vi "MeasurementGFV.vi"(8 "error in (no error)":errorcluster, 10 "MeasuremetnGFVEnum":T1=enum."Insert Single Measurement", 11 "Variant in":variant) -> (0 "error out":errorcluster, 3 "Variant Out":variant)   [LabVIEW 2013]
doc: "Use this template to build a VI to use as a subVI."
uses:
  Measurement Typedefs/MeasurementGFV.ctl
  General TypeDefs/MeasurementType.ctl
  General TypeDefs/ConfigurationDataTypeDef.ctl
  General TypeDefs/MeasurementDataType.ctl
  <vilib>/Utility/file.llb/Write To Spreadsheet File (string).vi
  Measurement Typedefs/KineticNotifierDatatype.ctl
panel:
  out "size(s)":i32
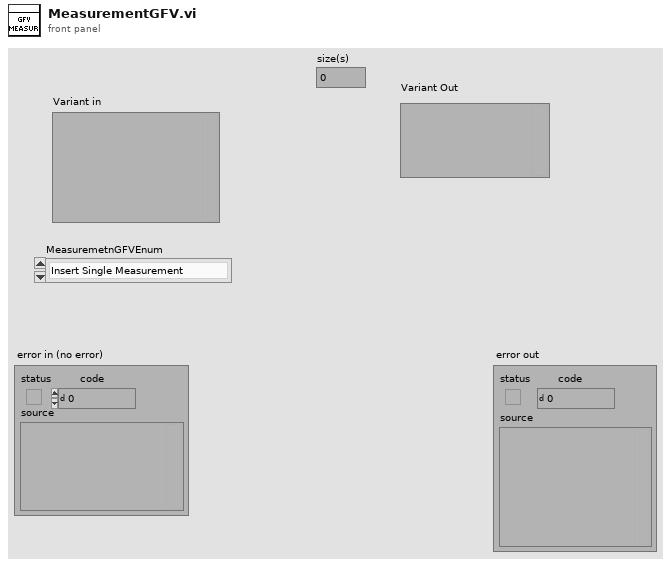
[diagram p1: front panel]
types:
  T1 = typedef "MeasurementGFV.ctl" = enum16{"Write 2 Excel", "Open Excel", "Close Excel", "Export To Excel", "GetExperimentGoalRemarks", "Load Single DB", "Save Single 2 DB", "Load Kinetic DB", "Save Kinetic 2 DB", "Get List of Wavelength", "Remove Wavelength", "Add Wavelength", "Get Sample Names", "Insert Sample Name", "Update Kinetic Display", "Update Single Display", "Init", "Insert General", "Init Single Measurement", "Insert Single Measurement", "Insert Kinetic Measurement", "Init Kinetic Measurment", "Init General"}
  T2 = typedef "MeasurementType.ctl" = enum16{"Single Meas", "Kinetic"}
  T3 = enum16{"open", "replace", "create", "open or create", "replace or create", "replace or create with confirmation"}
  T4 = typedef "ConfigurationDataTypeDef.ctl" = cluster{"Experiment Name":string, "File Path":path, "Goal":string, "Remarks":string, "Time Between Consecutive Frames (sec)":dbl, "Rq. No. of saves":i32, "Enable\nAutomatic\nStop":bool, "Measurement Type":T2, "File Name":string, "Choose Spectrometer":refnum<visa-resource-name>, "Integration time (ms)":i32, "Delay between measurements (ms) ":i32, "Offset in Wavlength (nm)":dbl}
  T5 = typedef "MeasurementDataType.ctl" = cluster{"Wavelength (nm)":dbl[], "Absorption":dbl[][], "Time":timestamp[], "Ref Spectrum":dbl[], "Dark Spectrum":dbl[], "Number of\nsamples to average":i32, "Measured Spectrum":dbl[][], "Sample Name":string[], "Selected Wavelengths":dbl[]}
  T6 = cluster{"General Data and Instrument Configuration":T4, "Kinetic Measurement":T5}
  T7 = cluster{"Absorption Saved Results":refnum<vi>, "Absorption @ wavelengths vs Time":refnum<vi>, "Selected Wavelengths":refnum<vi>}
  T8 = typedef "NI_Matrix.lvlib/RealMatrix.ctl" = dbl[][]
  T9 = cluster{"Experiment Name":string, "Goal":string, "Remarks":string, "File Path":path}
  T10 = cluster{"Wavelength (nm)":dbl[], "Absorption":dbl[]}
  T11 = cluster{"Wavelength (nm)":dbl[], "Absorption":dbl[]}[]
  T12 = typedef "KineticNotifierDatatype.ctl" = cluster{"Wavelength (nm)":dbl[], "Dark_spectrum":dbl[], "Meas_spectrum":dbl[], "Ref_spectrum":dbl[], "Absorption_spectrum":dbl[]}
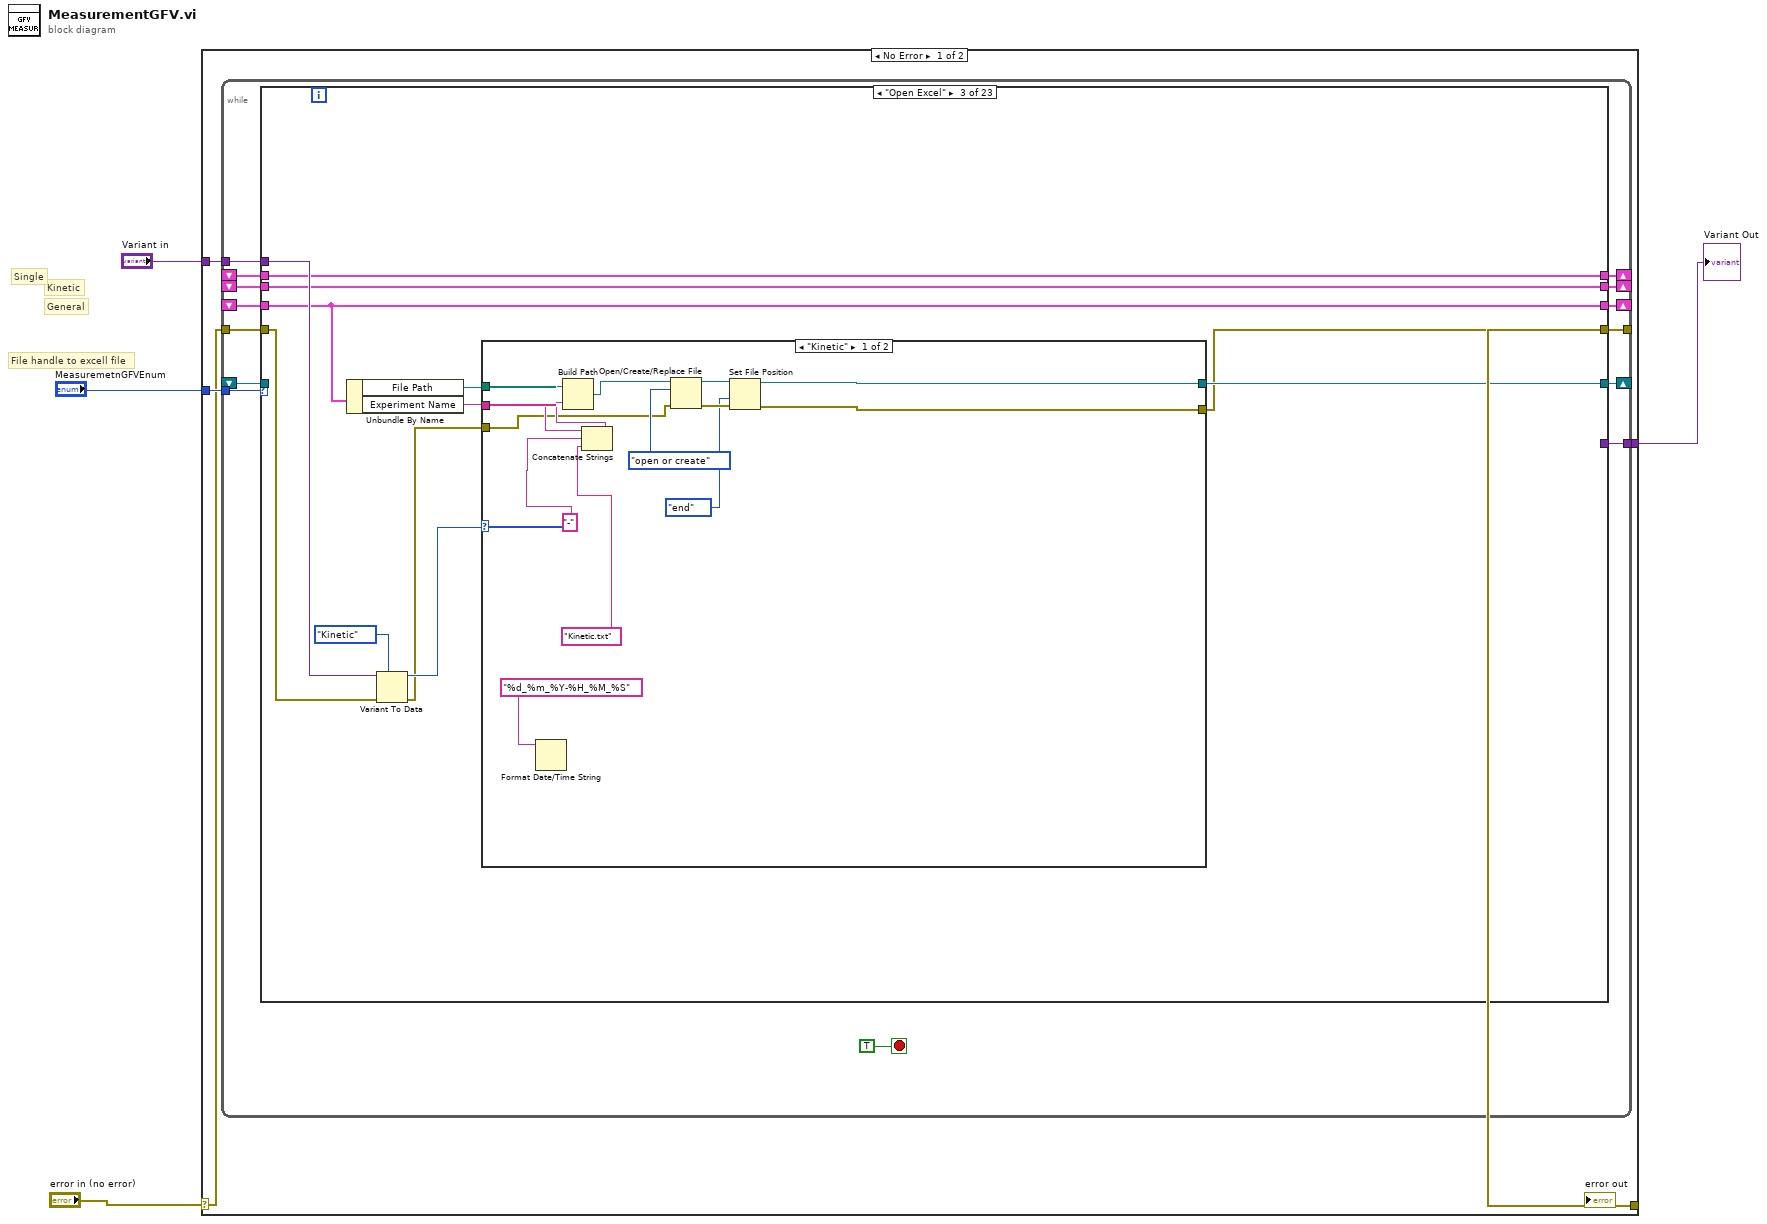
[diagram p0: block diagram]
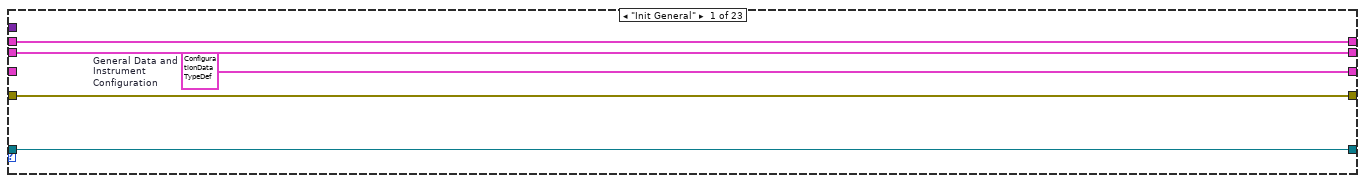
[diagram p2: hidden frame]
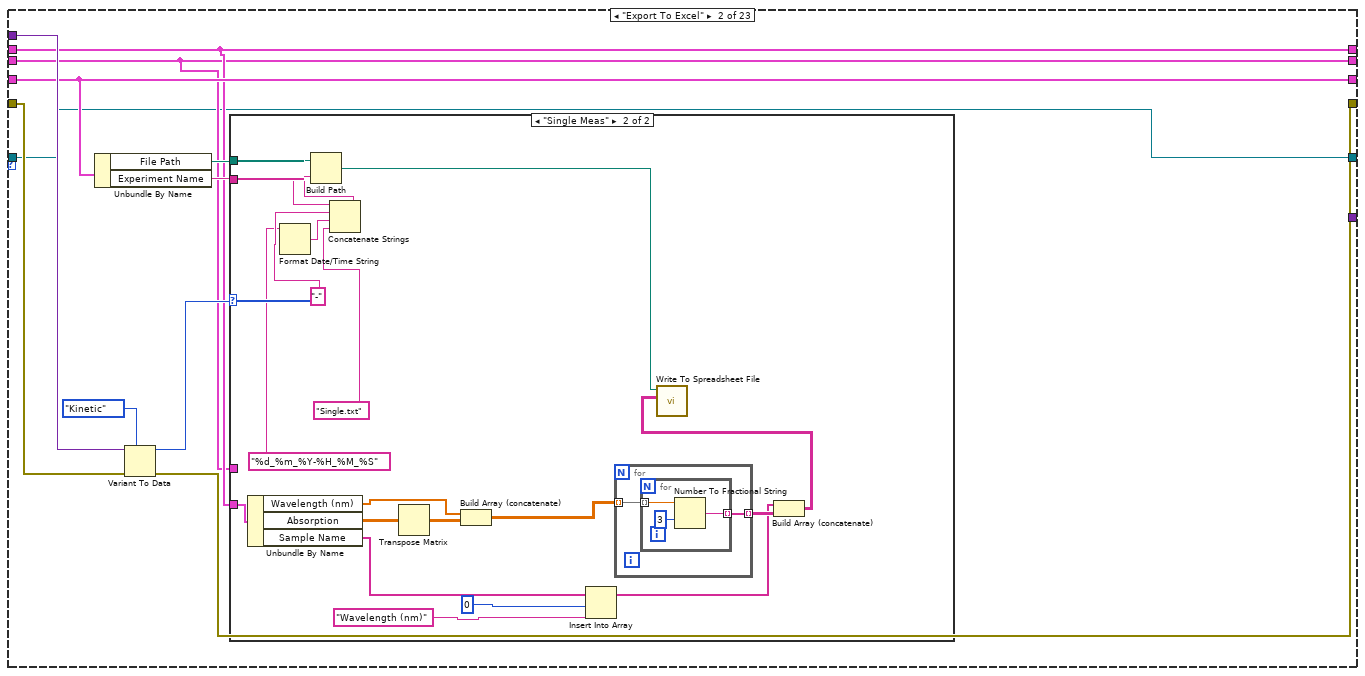
[diagram p3: hidden frame]
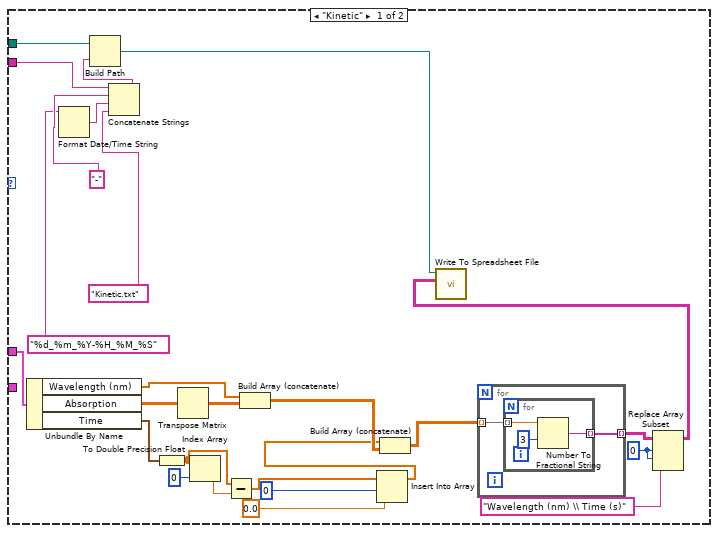
[diagram p4: hidden frame]
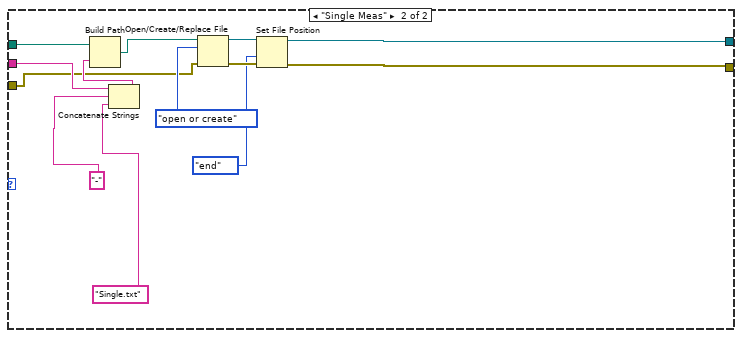
[diagram p5: hidden frame]
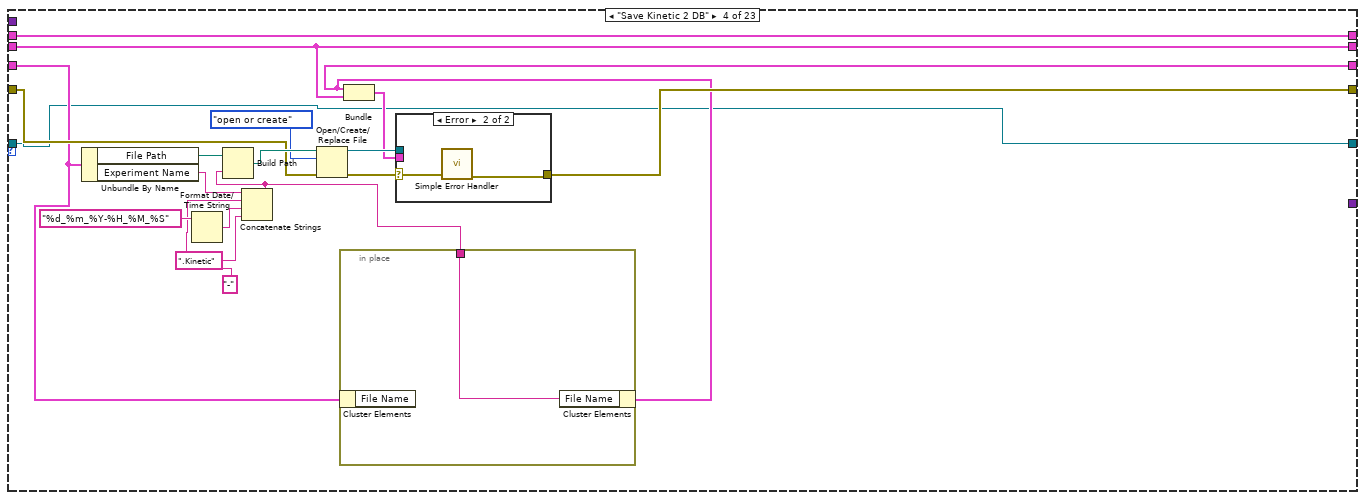
[diagram p6: hidden frame]
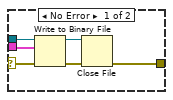
[diagram p7: hidden frame]
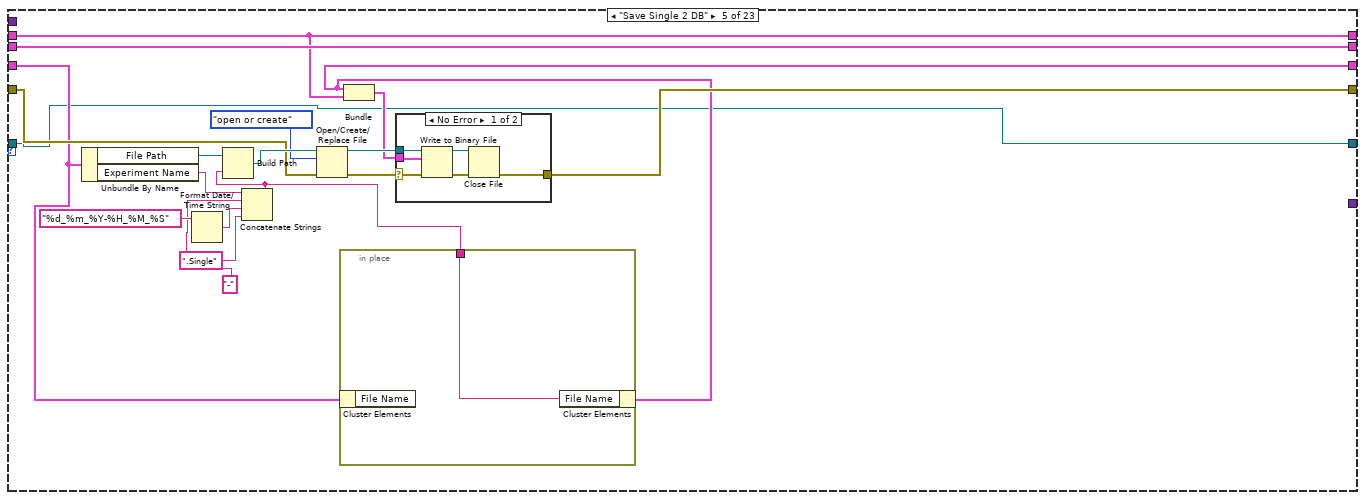
[diagram p8: hidden frame]
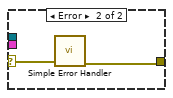
[diagram p9: hidden frame]
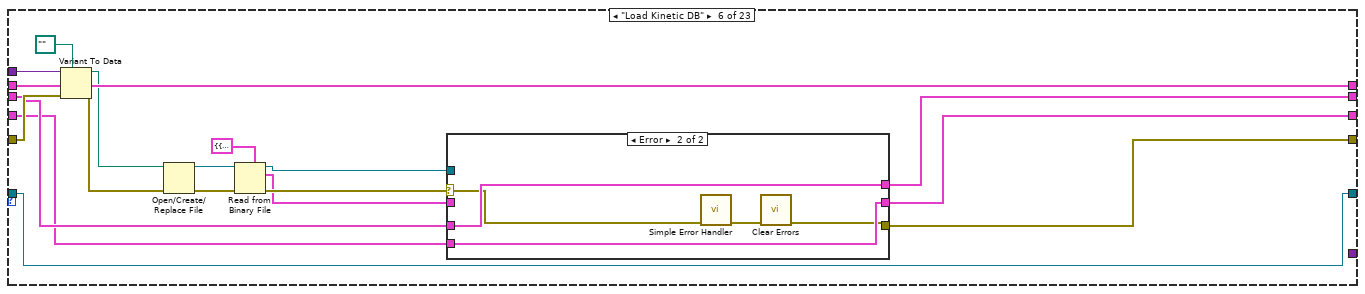
[diagram p10: hidden frame]
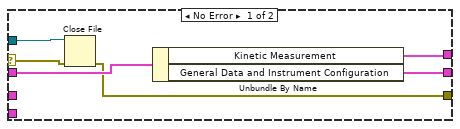
[diagram p11: hidden frame]
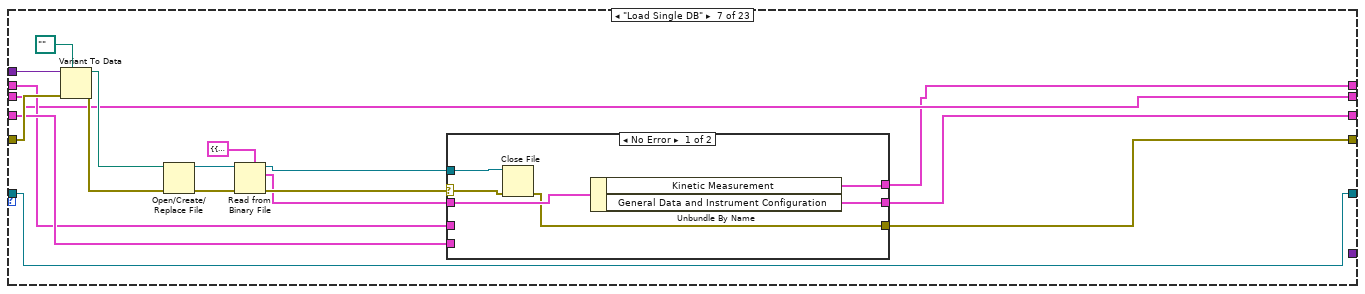
[diagram p12: hidden frame]
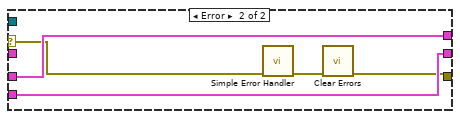
[diagram p13: hidden frame]
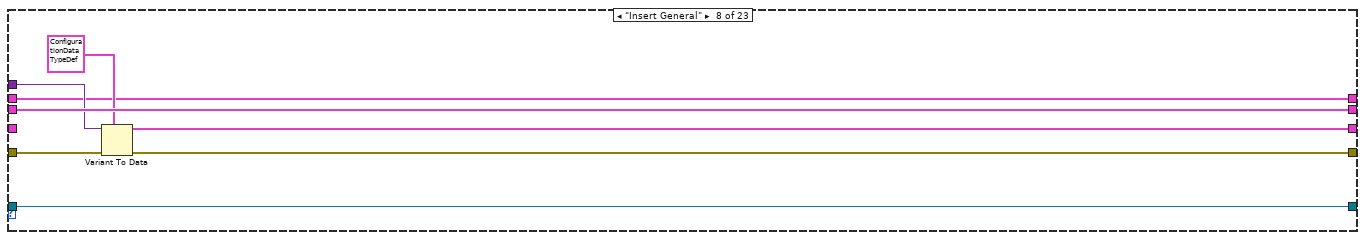
[diagram p14: hidden frame]
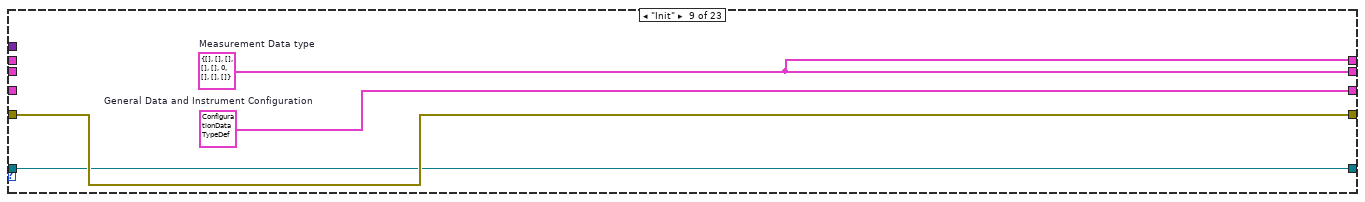
[diagram p15: hidden frame]
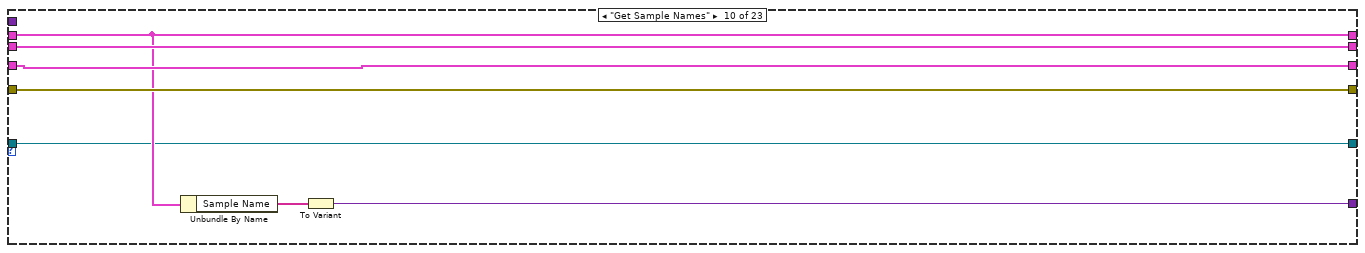
[diagram p16: hidden frame]
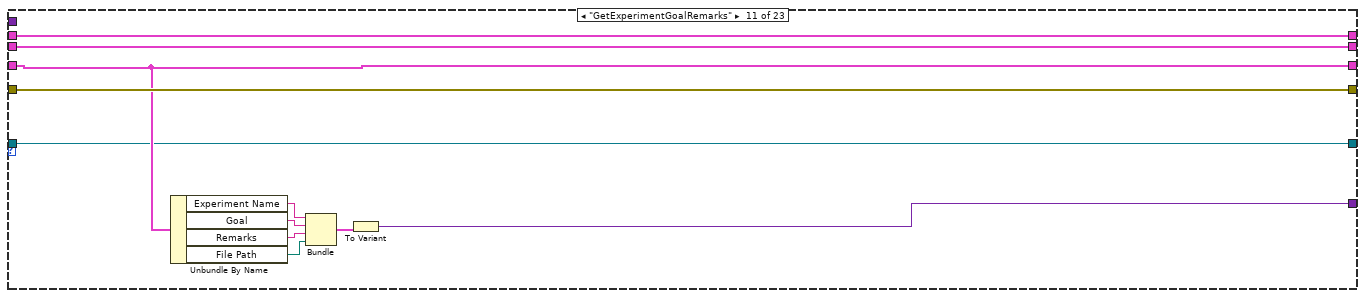
[diagram p17: hidden frame]
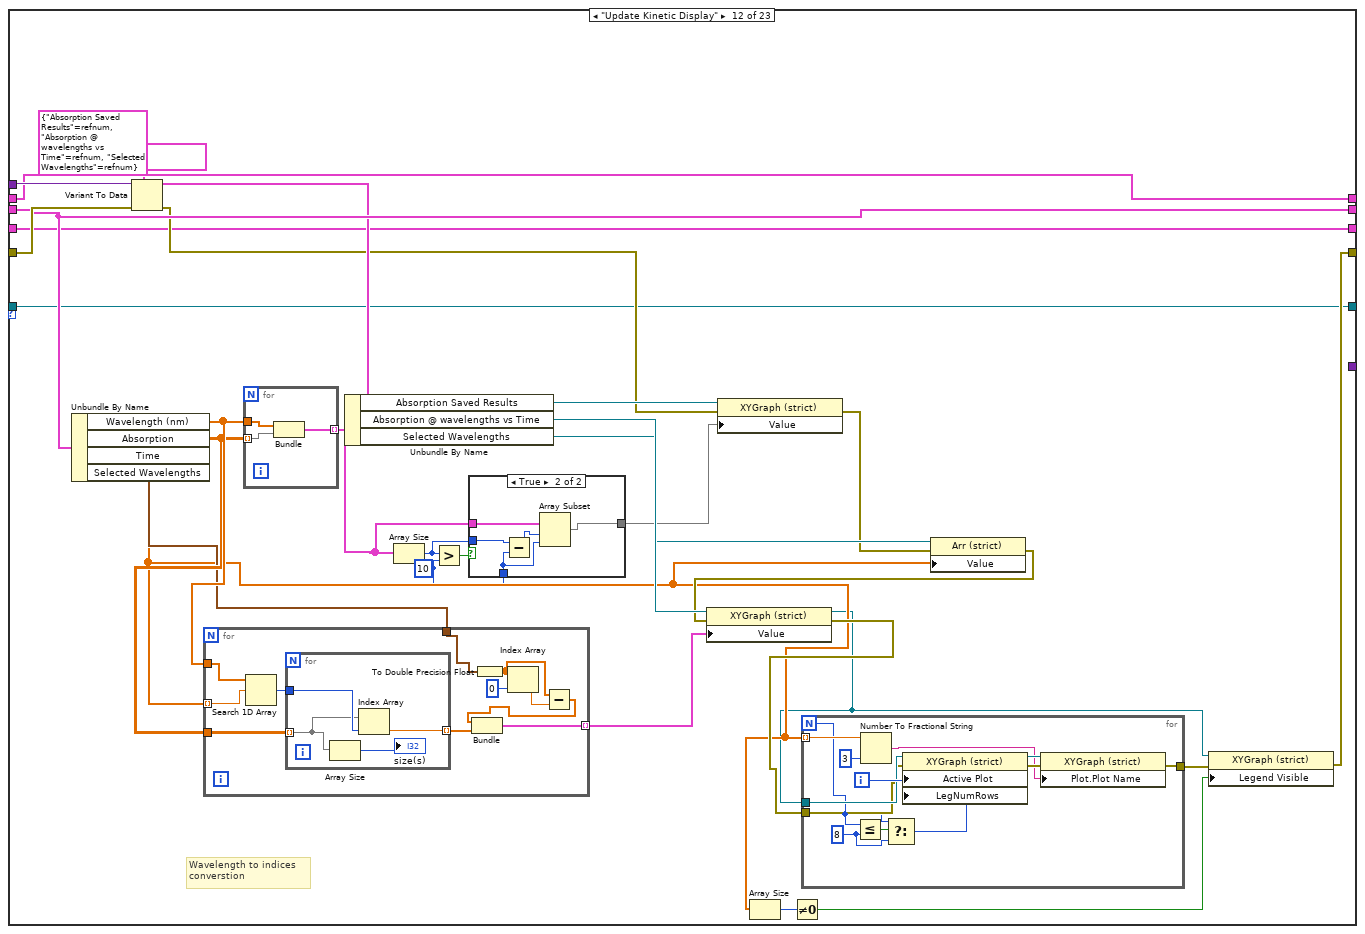
[diagram p18: hidden frame]
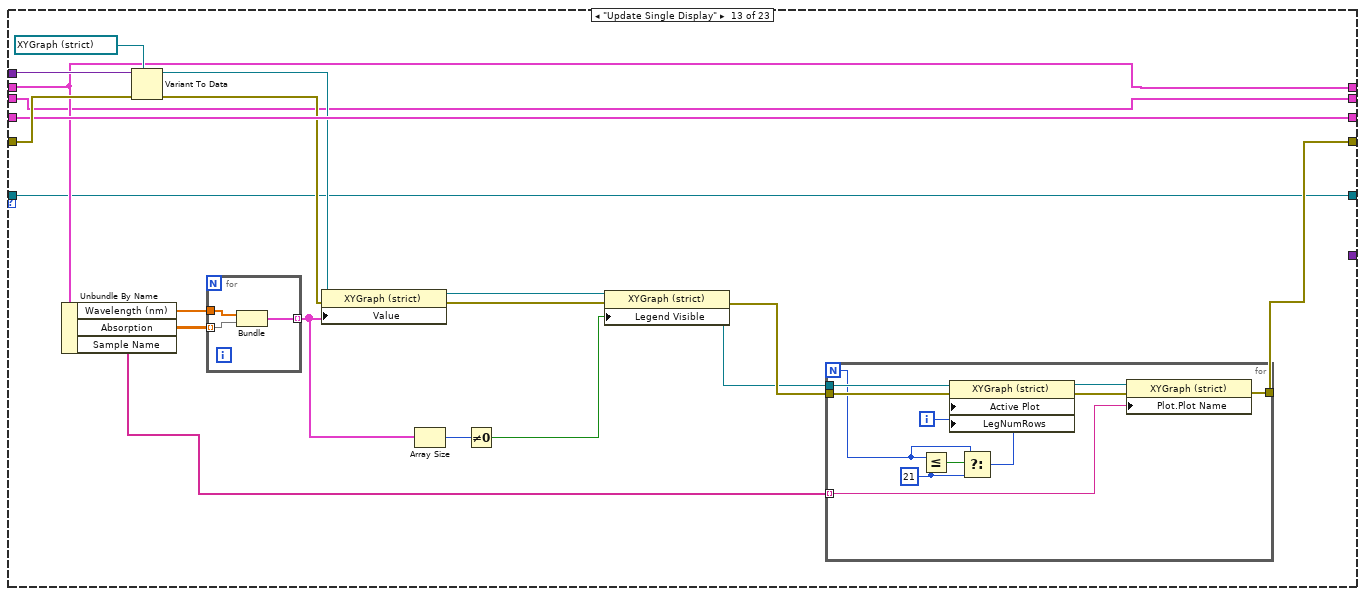
[diagram p20: hidden frame]
diagram:
  # "File handle to excell file"
  # "Single"
  # "General"
  # "Kinetic"
  n1 = case shown="No Error" "error in (no error)" {
    selector: "error in (no error)" -> [w8 w590]
    tunnel: [w7 w590] -> w4
    tunnel: "Variant in" -> [w10 _]
    tunnel: "MeasuremetnGFVEnum" -> [w9 _]
    tunnel: [w6 _] -> w1
    frame No Error {
      n2 = while {
        tunnel: w10 -> [w18]
        tunnel: w9 -> [w23]
        shift-right: [w22] -> _
        shift-left: _ -> [w20]
        shift-right: [w21] -> _
        shift-left: _ -> [w19]
        tunnel: w8 -> [w17]
        tunnel: [w16] -> w7
        shift-right: [w15] -> _
        shift-left: _ -> [w14]
        tunnel: [w13] -> w6
        shift-right: [w12] -> _
        shift-left: _ -> [w11]
        stop <- TRUE stop-if-true
        n3 = case shown="\"Open Excel\"" w23 {
          tunnel: [w28 w31 w99 w141 w170 w196 w222 w256 w258 w265 w277 w306 w355 w381 w396 w402 w415 w426 w447 w469 w478 w488 w490] -> w22
          tunnel: [w29 w37 w104 w136 w165 w195 w227 w253 w260 w266 w274 w296 w363 w389 w399 w401 w416 w432 w454 w474 w481 w487 w500] -> w21
          tunnel: w20 -> [w28 w31 w99 w141 w170 w193 w222 w256 _ w265 w277 w306 w355 w381 w396 w403 w414 w428 w447 w470 w478 w488 w490]
          tunnel: w19 -> [_ w37 w104 w138 w167 w192 w225 _ _ w266 w274 w296 w363 w389 w399 w401 w416 w432 w454 w474 w481 w487 w500]
          tunnel: w18 -> [_ w40 w107 _ _ w207 w237 w255 _ _ _ w308 w365 w388 _ w409 _ w429 w451 _ _ _ w498]
          tunnel: w17 -> [w27 w39 w106 w144 w173 w206 w236 w252 w259 w267 w278 w307 w364 w387 w397 w408 w417 w431 w453 w473 w480 w485 w497]
          tunnel: [w27 w33 w96 w142 w171 w194 w226 w251 w259 w267 w278 w285 w354 w386 w397 w407 w417 w431 w453 w473 w480 w482 w492] -> w16
          tunnel: [w26 w32 w100 w153 w164 w208 w221 w250 w258 w264 w276 w302 w356 w382 w398 w405 w418 w425 w448 w472 w479 w489 w491] -> w15
          tunnel: w14 -> [w26 w32 w100 w153 w164 w208 w223 w250 _ w264 w276 w302 w356 w383 w398 w405 w418 w425 w449 w472 _ w489 w491]
          tunnel: [_ _ _ _ _ _ _ _ _ w262 w275 _ _ _ w394 _ _ _ _ _ _ _ _] -> w13
          tunnel: [w25 w30 w98 w135 w163 w191 w220 w249 w257 w261 w269 w284 w346 w380 w393 w400 w413 w424 w446 w468 w477 refnum<file> refnum ("refnum out") w494] -> w12
          tunnel: w11 -> [w25 w30 _ w135 w163 w191 w220 w249 w257 w261 w269 w284 w346 w380 w393 w400 w413 w424 w446 w468 w477 w486 w495]
          frame "Init General" {
            w29 = T4 {"Experiment Name"="", "File Path"=path "E:/LINKAM Measurements_Naama", "Goal"="", "Remarks"="", "Time Between Consecutive Frames (sec)"=1.0, "Rq. No. of saves"=1, "Enable\nAutomatic\nStop"=TRUE, "Measurement Type"=enum."Single Meas", "File Name"="", "Choose Spectrometer"="USB650", "Integration time (ms)"=49, "Delay between measurements (ms) "=10, "Offset in Wavlength (nm)"=10.0}  # General Data and Instrument Configuration
          }
          frame "Export To Excel" {
            n4 = Unbundle By Name(w37) -> ("File Path"=w36:path, "Experiment Name"=w35:string)
            n5 = Variant To Data(error in=w39, type=MeasurementType."Kinetic" ("Measurement Type"), Variant=w40) -> (data=w34:T2, error out=w33:errorcluster)
            n6 = case shown="\"Single Meas\"" w34 {
              tunnel: w36 -> [w61 w85]
              tunnel: w35 -> [w60 w84]
              tunnel: w32 -> [_ w83]
              tunnel: w31 -> [w41 _]
              frame "Kinetic" {
                w44 = 0 ("index (row)")
                n7 = Unbundle By Name(w41) -> ("Wavelength (nm)"=w58:dbl[], "Absorption"=w59:dbl[][], "Time"=w52:timestamp[])
                n8 = Format Date/Time String(time format string (%c)="%d_%m_%Y-%H_%M_%S") -> (date/time string=w65:string)  [unwired: 2 in]
                n9 = Concatenate Strings(w60, "-" ("string"), w65, "Kinetic.txt" ("string")) -> (w66:string)
                n10 = Build Path(base path=w61, name or relative path=w66) -> (appended path=w56:path)
                n11 = To Double Precision Float(number=w52) -> (double precision float=w54:dbl[])
                n12 = Transpose Matrix(1:w59) -> (0:w57:dbl[][])
                n13 = Index Array(array=w54, index=0) -> (element=w53:dbl)
                n14 = Subtract(x=w54, y=w53) -> (x-y=w50:dbl[])
                n15 = Build Array (concatenate)(w58, w57) -> (w51:T8)
                n16 = Insert Into Array(array=w50, index=0, new element=0.0 ("new element/subarray")) -> (w47:dbl[])
                n17 = Build Array (concatenate)(w47, w51) -> (w46:T8)
                n18 = for {
                  tunnel: w46 -> [w68] mode=indexing
                  tunnel: [w67] -> w45 mode=indexing
                  n19 = for {
                    tunnel: w68 -> [w70] mode=indexing
                    tunnel: [w69] -> w67 mode=indexing
                    n20 = Number To Fractional String(number=w70, precision (6)=i16 3) -> (F-format string=w69:string)  [unwired: 2 in]
                  }
                }
                n21 = Replace Array Subset(array=w45, new element="Wavelength (nm) \\ Time (s)" ("new element/subarray"), index (row)=w44, index (col)=w44) -> (w42:string[][])
                n22 = call-poly <vilib>:"Write To Spreadsheet File.vi"("2D data"=w42, "file path (dialog if empty)"=w56) -> ()  [unwired: 6 in, 1 out]
              }
              frame "Single Meas" {
                n23 = Unbundle By Name(w83) -> ("Wavelength (nm)"=w81:dbl[], "Absorption"=w82:dbl[][], "Sample Name"=w77:string[])
                n24 = Format Date/Time String(time format string (%c)="%d_%m_%Y-%H_%M_%S") -> (date/time string=w89:string)  [unwired: 2 in]
                n25 = Concatenate Strings(w84, "-" ("string"), w89, "Single.txt" ("string")) -> (w90:string)
                n26 = Build Path(base path=w85, name or relative path=w90) -> (appended path=w79:path)
                n27 = Transpose Matrix(1:w82) -> (0:w80:dbl[][])
                n28 = Build Array (concatenate)(w81, w80) -> (w75:T8)
                n29 = Insert Into Array(array=w77, index=0, new element="Wavelength (nm)" ("new element/subarray")) -> (w73:string[])
                n30 = for {
                  tunnel: w75 -> [w92] mode=indexing
                  tunnel: [w91] -> w74 mode=indexing
                  n31 = for {
                    tunnel: w92 -> [w94] mode=indexing
                    tunnel: [w93] -> w91 mode=indexing
                    n32 = Number To Fractional String(number=w94, precision (6)=i16 3) -> (F-format string=w93:string)  [unwired: 2 in]
                  }
                }
                n33 = Build Array (concatenate)(w73, w74) -> (w72:string[][])
                n34 = call-poly <vilib>:"Write To Spreadsheet File.vi"("2D data"=w72, "file path (dialog if empty)"=w79) -> ()  [unwired: 6 in, 1 out]
              }
            }
          }
          frame "Open Excel" {
            n35 = Unbundle By Name(w104) -> ("File Path"=w103:path, "Experiment Name"=w102:string)
            n36 = Variant To Data(error in=w106, type=MeasurementType."Kinetic" ("Measurement Type"), Variant=w107) -> (data=w101:T2, error out=w97:errorcluster)
            n37 = case shown="\"Kinetic\"" w101 {
              tunnel: w103 -> [w118 w132]
              tunnel: w102 -> [w117 w131]
              tunnel: [w110 w124] -> w98
              tunnel: w97 -> [w111 w125]
              tunnel: [w109 w123] -> w96
              frame "Kinetic" {
                n38 = Format Date/Time String(time format string (%c)="%d_%m_%Y-%H_%M_%S") -> ()  [unwired: 2 in, 1 out]
                n39 = Concatenate Strings(w117, "-" ("string"), "Kinetic.txt" ("string")) -> (w121:string)
                n40 = Build Path(base path=w118, name or relative path=w121) -> (appended path=w116:path)
                n41 = Open/Create/Replace File(file path (use dialog)=w116, error in=w111, operation (0:open)=T3."open or create") -> (refnum out=w113:refnum<file>, error out=w114:errorcluster)  [unwired: 3 in, 1 out]
                n42 = Set File Position(refnum=w113, from (0:start)=enum16{"start", "end", "current"}."end", error in=w114) -> (refnum out=w110:refnum<file>, error out=w109:errorcluster)  [unwired: 1 in]
              }
              frame "Single Meas" {
                n43 = Concatenate Strings(w131, "-" ("string"), "Single.txt" ("string")) -> (w134:string)
                n44 = Build Path(base path=w132, name or relative path=w134) -> (appended path=w130:path)
                n45 = Open/Create/Replace File(file path (use dialog)=w130, error in=w125, operation (0:open)=T3."open or create") -> (refnum out=w127:refnum<file>, error out=w128:errorcluster)  [unwired: 3 in, 1 out]
                n46 = Set File Position(refnum=w127, from (0:start)=enum16{"start", "end", "current"}."end", error in=w128) -> (refnum out=w124:refnum<file>, error out=w123:errorcluster)  [unwired: 1 in]
              }
            }
          }
          frame "Save Kinetic 2 DB" {
            n47 = Unbundle By Name(w138) -> ("File Path"=w148:path, "Experiment Name"=w147:string)
            n48 = Format Date/Time String(time format string (%c)="%d_%m_%Y-%H_%M_%S") -> (date/time string=w150:string)  [unwired: 2 in]
            n49 = Concatenate Strings(w147, "-" ("string"), w150, ".Kinetic" ("string")) -> (w137:string)
            n50 = Build Path(base path=w148, name or relative path=w137) -> (appended path=w146:path)
            n51 = Open/Create/Replace File(file path (use dialog)=w146, error in=w144, operation (0:open)=T3."open or create") -> (refnum out=w143:refnum<file>, error out=w139:errorcluster)  [unwired: 3 in, 1 out]
            n52 = in-place {
              in-place-border: w137 -> [w154]
              n53 = in-place-cluster #1(w138) -> ()  [unwired: 1 out]
              n54 = in-place-cluster #1("File Name"=w154) -> (w136:T4)
            }
            n55 = Bundle("General Data and Instrument Configuration"=w136, "Kinetic Measurement"=w141) -> (w140:T6)  [unwired: 1 in]
            n56 = case shown="Error" w139 {
              selector: w139 -> [w155 w162]
              tunnel: w143 -> [w160 _]
              tunnel: [w157 w161] -> w142
              tunnel: w140 -> [w156 _]
              frame No Error {
                n57 = Write to Binary File(file (use dialog)=w160, data=w156, error in=w155) -> (refnum out=w158:refnum<file>, error out=w159:errorcluster)  [unwired: 3 in, 1 out]
                n58 = Close File(refnum=w158, error in=w159) -> (error out=w157:errorcluster)  [unwired: 1 out]
              }
              frame Error {
                n59 = call <vilib>:"Simple Error Handler.vi"("error in (no error)"=w162) -> ("error out"=w161:errorcluster)  [unwired: 4 in, 4 out]
              }
            }
          }
          frame "Save Single 2 DB" {
            n60 = Unbundle By Name(w167) -> ("File Path"=w177:path, "Experiment Name"=w176:string)
            n61 = Format Date/Time String(time format string (%c)="%d_%m_%Y-%H_%M_%S") -> (date/time string=w179:string)  [unwired: 2 in]
            n62 = Concatenate Strings(w176, "-" ("string"), w179, ".Single" ("string")) -> (w166:string)
            n63 = Build Path(base path=w177, name or relative path=w166) -> (appended path=w175:path)
            n64 = Open/Create/Replace File(file path (use dialog)=w175, error in=w173, operation (0:open)=T3."open or create") -> (refnum out=w172:refnum<file>, error out=w168:errorcluster)  [unwired: 3 in, 1 out]
            n65 = in-place {
              in-place-border: w166 -> [w182]
              n66 = in-place-cluster #2(w167) -> ()  [unwired: 1 out]
              n67 = in-place-cluster #2("File Name"=w182) -> (w165:T4)
            }
            n68 = Bundle("General Data and Instrument Configuration"=w165, "Kinetic Measurement"=w164) -> (w169:T6)  [unwired: 1 in]
            n69 = case shown="No Error" w168 {
              selector: w168 -> [w183 w190]
              tunnel: w172 -> [w188 _]
              tunnel: [w185 w189] -> w171
              tunnel: w169 -> [w184 _]
              frame No Error {
                n70 = Write to Binary File(file (use dialog)=w188, data=w184, error in=w183) -> (refnum out=w186:refnum<file>, error out=w187:errorcluster)  [unwired: 3 in, 1 out]
                n71 = Close File(refnum=w186, error in=w187) -> (error out=w185:errorcluster)  [unwired: 1 out]
              }
              frame Error {
                n72 = call <vilib>:"Simple Error Handler.vi"("error in (no error)"=w190) -> ("error out"=w189:errorcluster)  [unwired: 4 in, 4 out]
              }
            }
          }
          frame "Load Kinetic DB" {
            n73 = Variant To Data(error in=w206, type=path "" ("selected path"), Variant=w207) -> (data=w204:path, error out=w203:errorcluster)
            n74 = Open/Create/Replace File(file path (use dialog)=w204, error in=w203) -> (refnum out=w202:refnum<file>, error out=w201:errorcluster)  [unwired: 4 in, 1 out]
            n75 = Read from Binary File(5:T6 {"General Data and Instrument Configuration"={"Experiment Name"="", "File Path"=path "", "Goal"="", "Remarks"="", "Time Between Consecutive Frames (sec)"=0.0, "Rq. No. of saves"=0, "Enable\nAutomatic\nStop"=FALSE, "Measurement Type"=enum."Single Meas", "File Name"="", "Choose Spectrometer"="", "Integration time (ms)"=0, "Delay between measurements (ms) "=0, "Offset in Wavlength (nm)"=0.0}, "Kinetic Measurement"={"Wavelength (nm)"=[], "Absorption"=[], "Time"=[], "Ref Spectrum"=[], "Dark Spectrum"=[], "Number of\nsamples to average"=0, "Measured Spectrum"=[], "Sample Name"=[], "Selected Wavelengths"=[]}} ("output cluster"), 8:w201, 11:w202) -> (0:w199:errorcluster, 2:w197:T6, 3:w198:refnum<file>)  [unwired: 3 in, 1 out]
            n76 = case shown="Error" w199 {
              selector: w199 -> [w213 w216]
              tunnel: w198 -> [w214 _]
              tunnel: w197 -> [w212 _]
              tunnel: [w211 w219] -> w196
              tunnel: [w210 w218] -> w195
              tunnel: [w209 w215] -> w194
              tunnel: w193 -> [_ w219]
              tunnel: w192 -> [_ w218]
              frame No Error {
                n77 = Close File(refnum=w214, error in=w213) -> (error out=w209:errorcluster)  [unwired: 1 out]
                n78 = Unbundle By Name(w212) -> ("Kinetic Measurement"=w211:T5, "General Data and Instrument Configuration"=w210:T4)
              }
              frame Error {
                n79 = call <vilib>:"Simple Error Handler.vi"("error in (no error)"=w216) -> ("error out"=w217:errorcluster)  [unwired: 4 in, 4 out]
                n80 = call <vilib>:"Clear Errors.vi"("error in (no error)"=w217) -> ("error out"=w215:errorcluster)  [unwired: 6 in]
              }
            }
          }
          frame "Load Single DB" {
            n81 = Variant To Data(error in=w236, type=path "" ("selected path"), Variant=w237) -> (data=w234:path, error out=w233:errorcluster)
            n82 = Open/Create/Replace File(file path (use dialog)=w234, error in=w233) -> (refnum out=w232:refnum<file>, error out=w231:errorcluster)  [unwired: 4 in, 1 out]
            n83 = Read from Binary File(5:T6 {"General Data and Instrument Configuration"={"Experiment Name"="", "File Path"=path "", "Goal"="", "Remarks"="", "Time Between Consecutive Frames (sec)"=0.0, "Rq. No. of saves"=0, "Enable\nAutomatic\nStop"=FALSE, "Measurement Type"=enum."Single Meas", "File Name"="", "Choose Spectrometer"="", "Integration time (ms)"=0, "Delay between measurements (ms) "=0, "Offset in Wavlength (nm)"=0.0}, "Kinetic Measurement"={"Wavelength (nm)"=[], "Absorption"=[], "Time"=[], "Ref Spectrum"=[], "Dark Spectrum"=[], "Number of\nsamples to average"=0, "Measured Spectrum"=[], "Sample Name"=[], "Selected Wavelengths"=[]}} ("output cluster"), 8:w231, 11:w232) -> (0:w230:errorcluster, 2:w228:T6, 3:w229:refnum<file>)  [unwired: 3 in, 1 out]
            n84 = case shown="No Error" w230 {
              selector: w230 -> [w242 w245]
              tunnel: w229 -> [w243 _]
              tunnel: w228 -> [w241 _]
              tunnel: [w240 w248] -> w221
              tunnel: [w239 w247] -> w227
              tunnel: [w238 w244] -> w226
              tunnel: w223 -> [_ w248]
              tunnel: w225 -> [_ w247]
              frame No Error {
                n85 = Close File(refnum=w243, error in=w242) -> (error out=w238:errorcluster)  [unwired: 1 out]
                n86 = Unbundle By Name(w241) -> ("Kinetic Measurement"=w240:T5, "General Data and Instrument Configuration"=w239:T4)
              }
              frame Error {
                n87 = call <vilib>:"Simple Error Handler.vi"("error in (no error)"=w245) -> ("error out"=w246:errorcluster)  [unwired: 4 in, 4 out]
                n88 = call <vilib>:"Clear Errors.vi"("error in (no error)"=w246) -> ("error out"=w244:errorcluster)  [unwired: 6 in]
              }
            }
          }
          frame "Insert General" {
            n89 = Variant To Data(error in=w252, type=T4 {"Experiment Name"="", "File Path"=path "E:/LINKAM Measurements_Naama", "Goal"="", "Remarks"="", "Time Between Consecutive Frames (sec)"=1.0, "Rq. No. of saves"=1, "Enable\nAutomatic\nStop"=TRUE, "Measurement Type"=enum."Single Meas", "File Name"="", "Choose Spectrometer"="USB650", "Integration time (ms)"=49, "Delay between measurements (ms) "=10, "Offset in Wavlength (nm)"=10.0} ("General Data and Instrument Configuration"), Variant=w255) -> (data=w253:T4, error out=w251:errorcluster)
          }
          frame "Init" {
            w260 = T4 {"Experiment Name"="", "File Path"=path "E:/LINKAM Measurements_Naama", "Goal"="", "Remarks"="", "Time Between Consecutive Frames (sec)"=1.0, "Rq. No. of saves"=1, "Enable\nAutomatic\nStop"=TRUE, "Measurement Type"=enum."Single Meas", "File Name"="", "Choose Spectrometer"="USB650", "Integration time (ms)"=49, "Delay between measurements (ms) "=10, "Offset in Wavlength (nm)"=10.0}  # General Data and Instrument Configuration
            w258 = T5 {"Wavelength (nm)"=[], "Absorption"=[], "Time"=[], "Ref Spectrum"=[], "Dark Spectrum"=[], "Number of\nsamples to average"=0, "Measured Spectrum"=[], "Sample Name"=[], "Selected Wavelengths"=[]}  # Measurement Data type
          }
          frame "Get Sample Names" {
            n90 = Unbundle By Name(w264) -> ("Sample Name"=w263:string[])
            n91 = To Variant(anything=w263) -> (Variant=w262:variant)
          }
          frame "GetExperimentGoalRemarks" {
            n92 = Unbundle By Name(w274) -> ("Experiment Name"=w272:string, "Goal"=w271:string, "Remarks"=w270:string, "File Path"=w268:path)
            n93 = Bundle("Experiment Name"=w272, "Goal"=w271, "Remarks"=w270, "File Path"=w268) -> (w273:T9)  [unwired: 1 in]
            n94 = To Variant(anything=w273) -> (Variant=w275:variant)
          }
          frame "Update Kinetic Display" {
            w279 = 10 ("y")
            # "Wavelength to indices \nconverstion"
            n95 = Unbundle By Name(w306) -> ("Wavelength (nm)"=w300:dbl[], "Absorption"=w299:dbl[][], "Time"=w298:timestamp[], "Selected Wavelengths"=w289:dbl[])
            n96 = Variant To Data(error in=w307, type=T7 {"Absorption Saved Results"=refnum, "Absorption @ wavelengths vs Time"=refnum, "Selected Wavelengths"=refnum} ("output cluster"), Variant=w308) -> (data=w305:T7, error out=w303:errorcluster)
            n97 = for {
              tunnel: w289 -> [w333] mode=indexing
              tunnel: w300 -> [w338]
              tunnel: w299 -> [w337]
              tunnel: w298 -> [w332]
              tunnel: [w334] -> w297 mode=indexing
              n98 = Search 1D Array(1D array=w338, element=w333) -> (index of element=w336:i32)  [unwired: 1 in]
              n99 = for {
                tunnel: w337 -> [w340] mode=indexing
                tunnel: w336 -> [w342]
                tunnel: [w341] -> w335 mode=indexing
                n100 = Array Size(array=w340) -> (size(s)=→"size(s)":i32)
                n101 = Index Array(array=w340, index=w342) -> (element=w341:dbl)
              }
              n102 = To Double Precision Float(number=w332) -> (double precision float=w330:dbl[])
              n103 = Index Array(array=w330, index=0) -> (element=w329:dbl)
              n104 = Subtract(x=w330, y=w329) -> (x-y=w328:dbl[])
              n105 = Bundle(w328, w335) -> (w334:cluster{dbl[], dbl[]})  [unwired: 1 in]
            }
            n106 = for {
              tunnel: w299 -> [w344] mode=indexing
              tunnel: w300 -> [w345]
              tunnel: [w343] -> w282 mode=indexing
              n107 = Bundle("Wavelength (nm)"=w345, "Absorption"=w344) -> (w343:T10)  [unwired: 1 in]
            }
            n108 = Unbundle By Name(w305) -> ("Absorption Saved Results"=w304:refnum<vi>, "Absorption @ wavelengths vs Time"=w301:refnum<vi>, "Selected Wavelengths"=w294:refnum<vi>)
            n109 = Array Size(array=w282) -> (size(s)=w280:i32)
            n110 = Greater?(x=w280, y=w279) -> (0:w283:bool)
            n111 = case shown="True" w283 {
              tunnel: w282 -> [w309 w314]
              tunnel: [w309 w310] -> w281
              tunnel: w280 -> [_ w313]
              tunnel: w279 -> [_ w311]
              frame False {
              }
              frame True {
                n112 = Subtract(x=w313, y=w311) -> (x-y=w312:i32)
                n113 = Array Subset(array=w314, index=w312, length=w311) -> (w310:T11)
              }
            }
            n114 = property class="XYGraph (strict)"(reference=w304, error in=w303, "Value"=w281) -> (error out=w293:errorcluster)  [unwired: 1 out]
            n115 = Array Size(array=w289) -> (size(s)=w290:i32)
            n116 = Not Equal To 0?(x=w290) -> (x != 0?=w287:bool)
            n117 = property class="Arr (strict)"(reference=w294, error in=w293, "Value"=w289) -> (error out=w292:errorcluster)  [unwired: 1 out]
            n118 = property class="XYGraph (strict)"(reference=w301, error in=w292, "Value"=w297) -> (reference out=w286:refnum<vi>, error out=w291:errorcluster)
            n119 = for {
              N -> [w317]
              tunnel: w289 -> [w327] mode=indexing
              tunnel: w286 -> [w324]
              tunnel: w291 -> [w320]
              tunnel: [w319] -> w288
              i -> [w325]
              w316 = 8 ("y")
              n120 = Less Or Equal?(x=w317, y=w316) -> (x <= y?=w318:bool)
              n121 = Number To Fractional String(number=w327, precision (6)=i16 3) -> (F-format string=w321:string)  [unwired: 2 in]
              n122 = Select(t=w317, s=w318, f=w316) -> (s? t:f=w315:i32)
              n123 = property class="XYGraph (strict)"(reference=w324, error in=w320, "Active Plot"=w325, "LegNumRows"=w315) -> (reference out=w323:refnum<vi>, error out=w322:errorcluster)
              n124 = property class="XYGraph (strict)"(reference=w323, error in=w322, "Plot.Plot Name"=w321) -> (error out=w319:errorcluster)  [unwired: 1 out]
            }
            n125 = property class="XYGraph (strict)"(reference=w286, error in=w288, "Legend Visible"=w287) -> (error out=w285:errorcluster)  [unwired: 1 out]
          }
          frame "Update Single Display" {
            n126 = Unbundle By Name(w356) -> ("Wavelength (nm)"=w361:dbl[], "Absorption"=w362:dbl[][], "Sample Name"=w357:string[])
            n127 = Variant To Data(error in=w364, type=refnum<vi> refnum ("Absorption Saved Results"), Variant=w365) -> (data=w358:refnum<vi>, error out=w360:errorcluster)
            n128 = for {
              tunnel: w362 -> [w378] mode=indexing
              tunnel: w361 -> [w379]
              tunnel: [w377] -> w351 mode=indexing
              n129 = Bundle("Wavelength (nm)"=w379, "Absorption"=w378) -> (w377:T10)  [unwired: 1 in]
            }
            n130 = property class="XYGraph (strict)"(reference=w358, error in=w360, "Value"=w351) -> (reference out=w348:refnum<vi>, error out=w350:errorcluster)
            n131 = Array Size(array=w351) -> (size(s)=w353:i32)
            n132 = Not Equal To 0?(x=w353) -> (x != 0?=w352:bool)
            n133 = property class="XYGraph (strict)"(reference=w348, error in=w350, "Legend Visible"=w352) -> (reference out=w347:refnum<vi>, error out=w349:errorcluster)
            n134 = for {
              N -> [w366]
              tunnel: w347 -> [w376]
              tunnel: w357 -> [w371] mode=indexing
              tunnel: w349 -> [w374]
              tunnel: [w372] -> w354
              i -> [w368]
              w370 = 21 ("y")
              n135 = Less Or Equal?(x=w366, y=w370) -> (x <= y?=w369:bool)
              n136 = Select(t=w366, s=w369, f=w370) -> (s? t:f=w367:i32)
              n137 = property class="XYGraph (strict)"(reference=w376, error in=w374, "Active Plot"=w368, "LegNumRows"=w367) -> (reference out=w375:refnum<vi>, error out=w373:errorcluster)
              n138 = property class="XYGraph (strict)"(reference=w375, error in=w373, "Plot.Plot Name"=w371) -> (error out=w372:errorcluster)  [unwired: 1 out]
            }
          }
          frame "Insert Sample Name" {
            n139 = Variant To Data(error in=w387, type="" ("Sample Name"), Variant=w388) -> (data=w384:string, error out=w386:errorcluster)
            n140 = in-place {
              in-place-border: w384 -> [w390]
              n141 = in-place-cluster #3(w383) -> ("Sample Name"=w392:string[])
              n142 = Build Array (concatenate)(w392, w390) -> (w391:string[])
              n143 = in-place-cluster #3("Sample Name"=w391) -> (w382:T5)
            }
          }
          frame "Get List of Wavelength" {
            n144 = Unbundle By Name(w396) -> ("Selected Wavelengths"=w395:dbl[])
            n145 = To Variant(anything=w395) -> (Variant=w394:variant)
          }
          frame "Add Wavelength" {
            n146 = Variant To Data(error in=w408, type=0.0, Variant=w409) -> (data=w406:dbl, error out=w407:errorcluster)
            n147 = in-place {
              in-place-border: w406 -> [w410]
              n148 = in-place-cluster #4(w403) -> ("Selected Wavelengths"=w412:dbl[])
              n149 = Build Array (concatenate)(w412, w410) -> (w411:dbl[])
              n150 = in-place-cluster #4("Selected Wavelengths"=w411) -> (w402:T5)
            }
          }
          frame "Remove Wavelength" {
            n151 = in-place {
              n152 = in-place-cluster #5(w414) -> ("Selected Wavelengths"=w419:dbl[])
              n153 = Array Size(array=w419) -> (size(s)=w422:i32)
              n154 = Decrement(x=w422) -> (x-1=w421:i32)
              n155 = Delete From Array(array=w419, length=1, index=w421) -> (array with subset deleted=w420:dbl[])  [unwired: 1 out]
              n156 = in-place-cluster #5("Selected Wavelengths"=w420) -> (w415:T5)
            }
          }
          frame "Insert Kinetic Measurement" {
            w430 = T12 {"Wavelength (nm)"=[], "Dark_spectrum"=[], "Meas_spectrum"=[], "Ref_spectrum"=[], "Absorption_spectrum"=[]}  # KineticNotifierDataType
            n157 = Variant To Data(type=w430, Variant=w429) -> (data=w427:T12)  [unwired: 1 in, 1 out]
            n158 = in-place {
              in-place-border: [w445] -> _
              in-place-border: w427 -> [w445]
              n159 = in-place-cluster #6(w428) -> ("Measured Spectrum"=w441:dbl[][], "Absorption"=w437:dbl[][], "Time"=w435:timestamp[])  [unwired: 3 out]
              n160 = Unbundle By Name(w445) -> ("Wavelength (nm)"=w444:dbl[], "Ref_spectrum"=w443:dbl[], "Dark_spectrum"=w442:dbl[], "Meas_spectrum"=w440:dbl[], "Absorption_spectrum"=w436:dbl[])
              n161 = Get Date/Time In Seconds() -> (seconds since 1Jan1904=w434:timestamp)
              n162 = Build Array (concatenate)(w435, w434) -> (w433:timestamp[])
              n163 = Build Array (concatenate)(w441, w440) -> (w439:dbl[][])
              n164 = Build Array (concatenate)(w437, w436) -> (w438:dbl[][])
              n165 = in-place-cluster #6("Wavelength (nm)"=w444, "Ref Spectrum"=w443, "Dark Spectrum"=w442, "Measured Spectrum"=w439, "Absorption"=w438, "Time"=w433) -> (w426:T5)
            }
          }
          frame "Insert Single Measurement" {
            w452 = T12 {"Wavelength (nm)"=[], "Dark_spectrum"=[], "Meas_spectrum"=[], "Ref_spectrum"=[], "Absorption_spectrum"=[]}  # KineticNotifierDataType
            n166 = Variant To Data(type=w452, Variant=w451) -> (data=w450:T12)  [unwired: 1 in, 1 out]
            n167 = in-place {
              in-place-border: [w467] -> _
              in-place-border: w450 -> [w467]
              n168 = in-place-cluster #7(w449) -> ("Measured Spectrum"=w463:dbl[][], "Absorption"=w459:dbl[][], "Time"=w457:timestamp[])  [unwired: 3 out]
              n169 = Unbundle By Name(w467) -> ("Wavelength (nm)"=w466:dbl[], "Ref_spectrum"=w465:dbl[], "Dark_spectrum"=w464:dbl[], "Meas_spectrum"=w462:dbl[], "Absorption_spectrum"=w458:dbl[])
              n170 = Get Date/Time In Seconds() -> (seconds since 1Jan1904=w456:timestamp)
              n171 = Build Array (concatenate)(w457, w456) -> (w455:timestamp[])
              n172 = Build Array (concatenate)(w463, w462) -> (w461:dbl[][])
              n173 = Build Array (concatenate)(w459, w458) -> (w460:dbl[][])
              n174 = in-place-cluster #7("Wavelength (nm)"=w466, "Ref Spectrum"=w465, "Dark Spectrum"=w464, "Measured Spectrum"=w461, "Absorption"=w460, "Time"=w455) -> (w448:T5)
            }
          }
          frame "Init Kinetic Measurment" {
            w471 = T5 {"Wavelength (nm)"=[], "Absorption"=[], "Time"=[], "Ref Spectrum"=[], "Dark Spectrum"=[], "Number of\nsamples to average"=0, "Measured Spectrum"=[], "Sample Name"=[], "Selected Wavelengths"=[]}  # Kinetic Measurement
            n175 = in-place {
              in-place-border: w470 -> [w476]
              n176 = in-place-cluster #8(w471) -> ()  [unwired: 1 out]
              n177 = Unbundle By Name(w476) -> ("Selected Wavelengths"=w475:dbl[])
              n178 = in-place-cluster #8("Selected Wavelengths"=w475) -> (w469:T5)
            }
          }
          frame "Init Single Measurement" {
            w479 = T5 {"Wavelength (nm)"=[], "Absorption"=[], "Time"=[], "Ref Spectrum"=[], "Dark Spectrum"=[], "Number of\nsamples to average"=0, "Measured Spectrum"=[], "Sample Name"=[], "Selected Wavelengths"=[]}  # Kinetic Measurement
          }
          frame "Close Excel" {
            n179 = Close File(refnum=w486, error in=w485) -> (error out=w483:errorcluster)  [unwired: 1 out]
            n180 = call <vilib>:"Clear Errors.vi"("error in (no error)"=w483) -> ("error out"=w482:errorcluster)  [unwired: 6 in]
          }
          frame "Write 2 Excel" {
            n181 = Variant To Data(error in=w497, type=MeasurementType."Kinetic" ("Measurement Type"), Variant=w498) -> (data=w496:T2, error out=w493:errorcluster)
            n182 = case shown="\"Single Meas\"" w496 {
              tunnel: w495 -> [w513 w557]
              tunnel: [w503 w548] -> w494
              tunnel: w491 -> [_ w567]
              tunnel: w493 -> [w512 w556]
              tunnel: [w505 w550] -> w492
              tunnel: w490 -> [w502 _]
              frame "Kinetic" {
                n183 = Unbundle By Name(w502) -> ("Absorption"=w517:dbl[][], "Time"=w520:timestamp[], "Wavelength (nm)"=w501:dbl[])
                n184 = Matrix Size(0:w517) -> (1:w519:i32)  [unwired: 1 out]
                n185 = Equal?(x=w519, y=1) -> (x = y?=w522:bool)
                n186 = case shown="False" w522 {
                  tunnel: w513 -> [w530 w537]
                  tunnel: w512 -> [w529 w538]
                  tunnel: [w530 w535] -> w511
                  tunnel: [w529 w534] -> w510
                  tunnel: w501 -> [_ w531]
                  frame False {
                  }
                  frame True {
                    # "Write the first line"
                    n187 = for {
                      tunnel: w531 -> [w544] mode=indexing
                      tunnel: [w542] -> w540 mode=indexing
                      n188 = Number To Fractional String(number=w544, precision (6)=i16 3) -> (F-format string=w543:string)  [unwired: 2 in]
                      n189 = Concatenate Strings(w543, "\t") -> (w542:string)
                    }
                    n190 = Concatenate Strings("Time/Wavelength (nm)" ("string"), "\t", w540, "\r") -> (w536:string)
                    n191 = Write to Text File(file (use dialog)=w537, text=w536, error in=w538) -> (refnum out=w535:refnum<file>, error out=w534:errorcluster)  [unwired: 1 in, 1 out]
                  }
                }
                n192 = Decrement(x=w519) -> (x-1=w516:i32)
                n193 = Index Array(array=w517, index (row)=w516) -> (element=w515:dbl[])  [unwired: 1 in]
                n194 = Index Array(array=w520, index=w516) -> (element=w521:timestamp)
                n195 = Format Date/Time String(seconds (now)=w521) -> (date/time string=w508:string)  [unwired: 2 in]
                n196 = for {
                  tunnel: [w525] -> w518 mode=indexing
                  tunnel: w515 -> [w527] mode=indexing
                  n197 = Number To Fractional String(number=w527, precision (6)=i16 3) -> (F-format string=w526:string)  [unwired: 2 in]
                  n198 = Concatenate Strings(w526, "\t") -> (w525:string)
                }
                n199 = Concatenate Strings(w508, "\t", w518, "\r") -> (w514:string)
                n200 = Write to Text File(file (use dialog)=w511, text=w514, error in=w510) -> (refnum out=w504:refnum<file>, error out=w506:errorcluster)  [unwired: 1 in, 1 out]
                n201 = Flush File(refnum=w504, error in=w506) -> (refnum out=w503:refnum<file>, error out=w505:errorcluster)
              }
              frame "Single Meas" {
                n202 = Unbundle By Name(w567) -> ("Absorption"=w561:dbl[][], "Sample Name"=w564:string[], "Wavelength (nm)"=w546:dbl[])
                n203 = Matrix Size(0:w561) -> (1:w563:i32)  [unwired: 1 out]
                n204 = Equal?(x=w563, y=1) -> (x = y?=w565:bool)
                n205 = case shown="True" w565 {
                  tunnel: w557 -> [w574 w581]
                  tunnel: w556 -> [w573 w582]
                  tunnel: [w574 w579] -> w555
                  tunnel: [w573 w578] -> w554
                  tunnel: w546 -> [_ w575]
                  frame False {
                  }
                  frame True {
                    # "Write the first line"
                    n206 = for {
                      tunnel: w575 -> [w588] mode=indexing
                      tunnel: [w586] -> w584 mode=indexing
                      n207 = Number To Fractional String(number=w588, precision (6)=i16 3) -> (F-format string=w587:string)  [unwired: 2 in]
                      n208 = Concatenate Strings(w587, "\t") -> (w586:string)
                    }
                    n209 = Concatenate Strings("Sample Name/Wavelength (nm)" ("string"), "\t", w584, "\r") -> (w580:string)
                    n210 = Write to Text File(file (use dialog)=w581, text=w580, error in=w582) -> (refnum out=w579:refnum<file>, error out=w578:errorcluster)  [unwired: 1 in, 1 out]
                  }
                }
                n211 = Decrement(x=w563) -> (x-1=w560:i32)
                n212 = Index Array(array=w561, index (row)=w560) -> (element=w559:dbl[])  [unwired: 1 in]
                n213 = Index Array(array=w564, index=w560) -> (element=w547:string)
                n214 = for {
                  tunnel: [w569] -> w562 mode=indexing
                  tunnel: w559 -> [w571] mode=indexing
                  n215 = Number To Fractional String(number=w571, precision (6)=i16 3) -> (F-format string=w570:string)  [unwired: 2 in]
                  n216 = Concatenate Strings(w570, "\t") -> (w569:string)
                }
                n217 = Concatenate Strings(w547, "\t", w562, "\r") -> (w558:string)
                n218 = Write to Text File(file (use dialog)=w555, text=w558, error in=w554) -> (refnum out=w549:refnum<file>, error out=w551:errorcluster)  [unwired: 1 in, 1 out]
                n219 = Flush File(refnum=w549, error in=w551) -> (refnum out=w548:refnum<file>, error out=w550:errorcluster)
              }
            }
          }
        }
      }
    }
    frame Error {
    }
  }
  "error out" <- w4
  "Variant Out" <- w1
